vi "Parse Accelerometer ERD.vi"(0 "string":string) -> (14 "Peak Magnitude":dbl, 15 "Peak Signal":u8, 16 "Peak Direction":bool, 17 "Peak Vector":dbl)   [LabVIEW 2021]
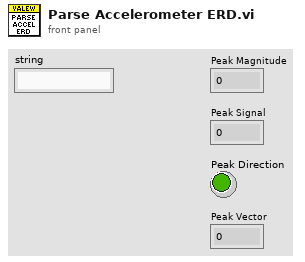
[diagram p1: front panel]
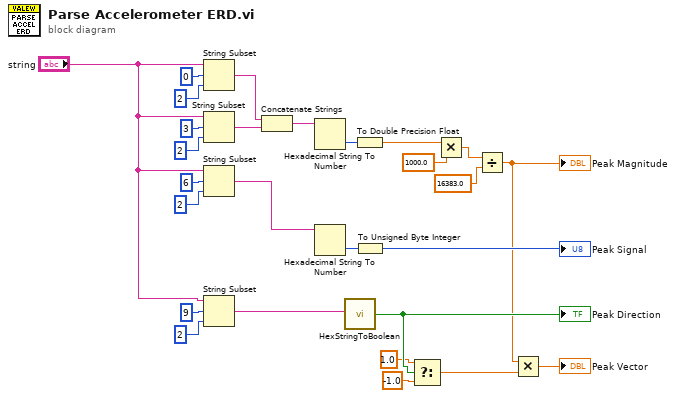
[diagram p0: block diagram]
diagram:
  n1 = String Subset(string="string", offset (0)=0, length (rest)=2 ("length (rest)")) -> (substring=w17:string)
  n2 = String Subset(string="string", offset (0)=3, length (rest)=2 ("length (rest)")) -> (substring=w16:string)
  n3 = String Subset(string="string", offset (0)=6, length (rest)=2 ("length (rest)")) -> (substring=w13:string)
  n4 = String Subset(string="string", offset (0)=9, length (rest)=2 ("length (rest)")) -> (substring=w11:string)
  n5 = Concatenate Strings(w17, w16) -> (w18:string)
  n6 = Hexadecimal String To Number(string=w18) -> (number=w15:u32)  [unwired: 2 in, 1 out]
  n7 = Hexadecimal String To Number(string=w13) -> (number=w14:u32)  [unwired: 2 in, 1 out]
  n8 = call "HexStringToBoolean.vi"("Hex String"=w11) -> ("Boolean"=w10:bool)
  "Peak Direction" <- w10
  n9 = To Double Precision Float(number=w15) -> (double precision float=w2:dbl)
  n10 = To Unsigned Byte Integer(number=w14) -> (unsigned 8bit integer=→"Peak Signal":u8)
  n11 = Select(t=1.0, s=w10, f=-1.0) -> (s? t:f=w7:dbl)
  n12 = Multiply(x=w2, y=1000.0) -> (x*y=w4:dbl)
  n13 = Divide(x=w4, y=16383.0) -> (x/y=w1:dbl)
  "Peak Magnitude" <- w1
  n14 = Multiply(x=w1, y=w7) -> (x*y=→"Peak Vector":dbl)
